vi "NewAutoRoutineCreator.vi"() -> ()   [LabVIEW 2017]
uses:
  Global.vi
  <vilib>/xml/Close Reference(Node).vi
  <resource>/objmgr/DOMUserDefRef.rc
  <vilib>/xml/NI_XML.lvlib
panel:
  out "Array":string[](array[string])
  out "XML":string
  out "Parse Errors":string
  in  "XML File Path":path=path "C:/Users/Bendethic/Desktop/AutoRoutineCreator/Test.txt"
  in  "Commands":i32(listbox)
  # "<Parallel>\n\t\t<Sequential>\n\t\t\t<DriveForTime speed=\"-0.4\" time=\"0.5\"/>\n\t\t\t<TurnToAngle angle=\"170\"/>\n\t\t</Sequential>\n\t\t<Sequential>\n\t\t\t<Wait time=\"0.3\"/>\n\t\t\t<RaiseElevator height=\"8\"/>\t\n\t\t</Sequential>\n\t</Parallel>\n\t<Parallel>\n\t\t<DriveForDistance speed=\"0.7\" distance=\"40\"/>\n\t\t<Intake speed=\"1\" time = \"3\" waitFor = \"false\"/>\n\t</Parallel>"
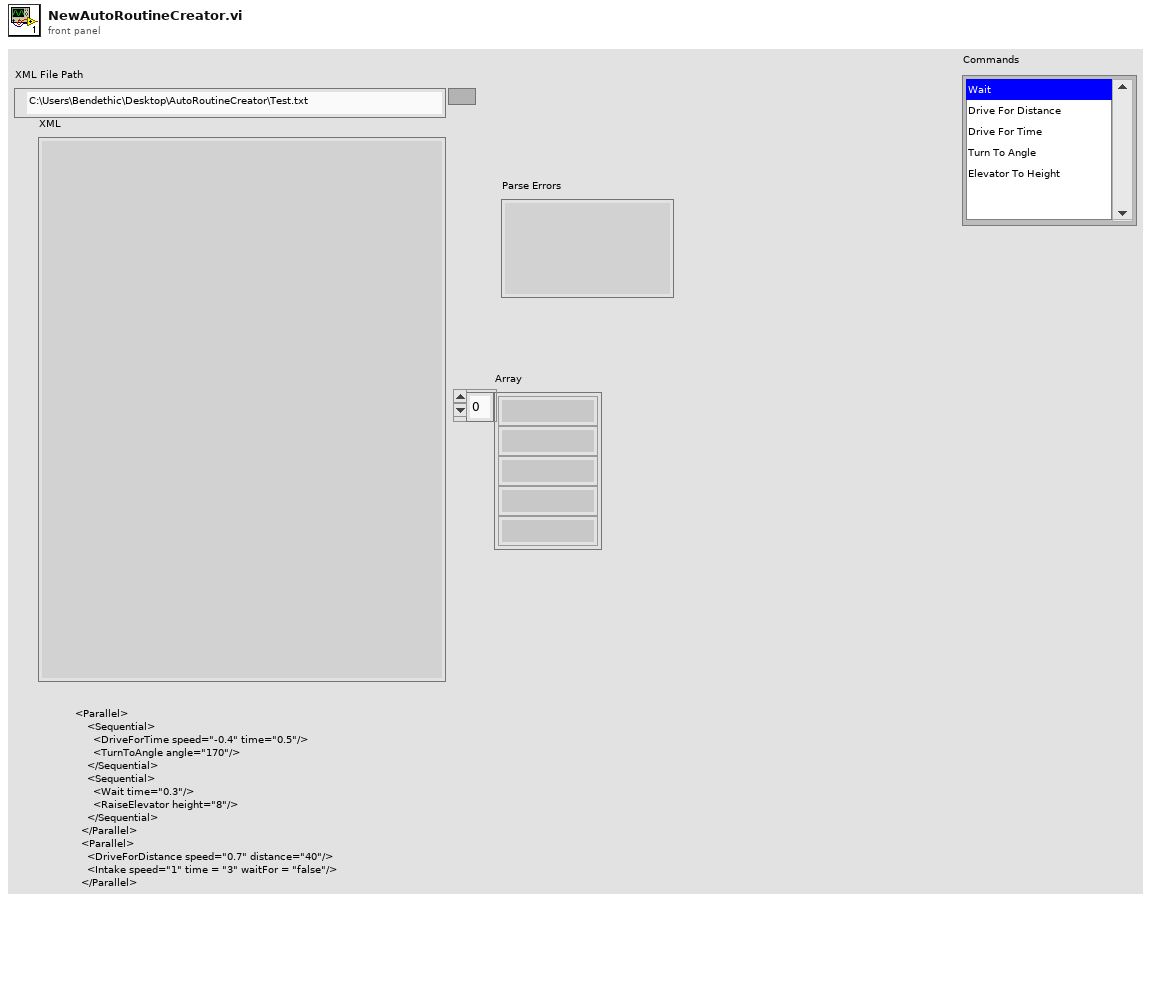
[diagram p1: front panel]
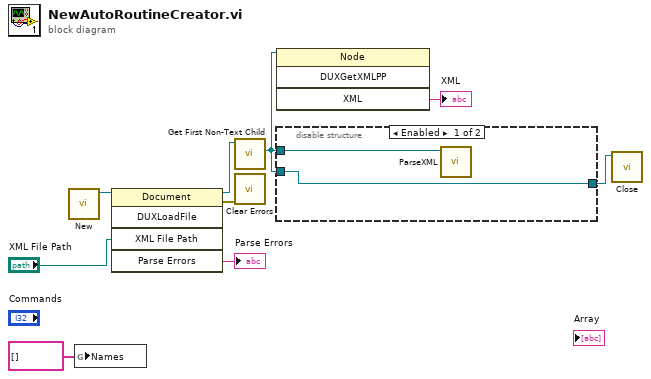
[diagram p0: block diagram]
diagram:
  n1 = call <vilib>:"New.vi"() -> ("DOM document out"=w7:refnum<k20>)  [unwired: 8 in, 1 out]
  n2 = global write "Global.vi" "Names"(string[] [] ("Names")) -> ()
  n3 = invoke class="Document" method="DUXLoadFile"(reference=w7, "XML File Path"="XML File Path") -> (reference out=w4:refnum<k20>, error out=w6:errorcluster, "Parse Errors"=→"Parse Errors":string)  [unwired: 3 in, 2 out]
  n4 = call <vilib>:"Get First Non-Text Child.vi"("node in"=w4) -> ("child node"=w2:refnum<k20>)  [unwired: 7 in, 3 out]
  n5 = call <vilib>:"Clear Errors.vi"("error in (no error)"=w6) -> ()  [unwired: 5 in, 2 out]
  n6 = invoke class="Node" method="DUXGetXMLPP"(reference=w2) -> ("XML"=→"XML":string)  [unwired: 3 in, 3 out]
  n7 = disable-structure shown="Enabled" {
    disable-tunnel: w2 -> [w11 _]
    disable-tunnel: w2 -> [w10 _]
    disable-tunnel: [w10 _] -> w1
    frame Enabled {
      n8 = call "ParseXML.vi"("Node"=w11) -> ()  [unwired: 10 in, 1 out]
    }
    frame Disabled {
    }
  }
  n9 = call-poly <vilib>:"Close.vi"("node"=w1) -> ()  [unwired: 8 in, 1 out]
